vi "Update_WebsocketConnection.vi"(7 "simple_html_chat_ui in":refnum<class "simple_html_chat_ui.lvclass">, 8 "error in (no error)":errorcluster, 11 "WebSocket Connection in":refnum<class "WebSocket Server.lvclass">) -> (0 "error out":errorcluster, 3 "WebSocket Connection out":refnum<class "WebSocket Server.lvclass">, 5 "simple_html_chat_ui out":refnum<class "simple_html_chat_ui.lvclass">)   [LabVIEW 2020, in "simple_html_chat_ui.lvclass"]
uses:
  simple_html_chat_ui.lvclass
  WebSockets-API/Source/WebSockets/WebSocket Server/WebSocket Server.lvclass
  ui/View.vi
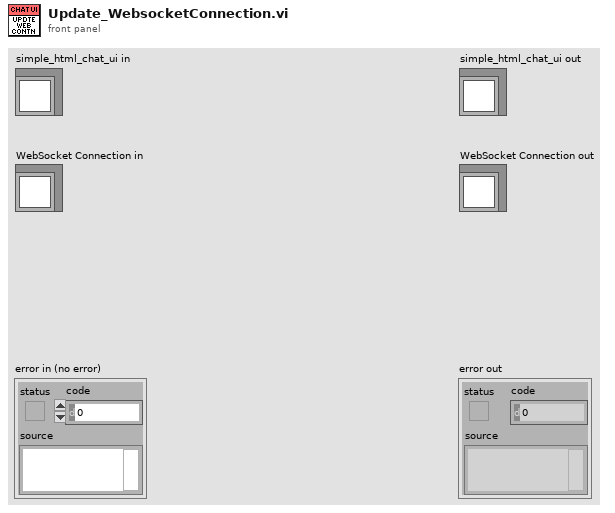
[diagram p1: front panel]
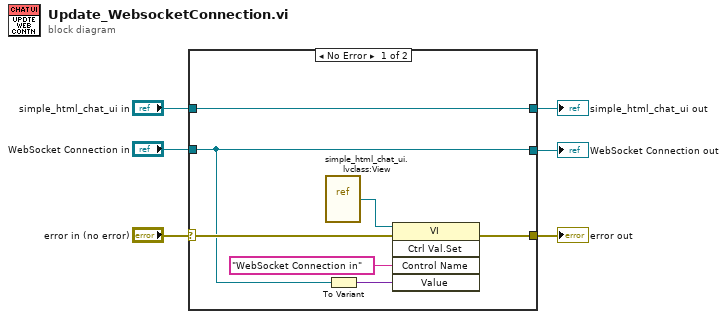
[diagram p0: block diagram]
diagram:
  n1 = case shown="No Error" "error in (no error)" {
    selector: "error in (no error)" -> [w9 w16]
    tunnel: [w8 w16] -> w5
    tunnel: [w13 w15] -> w3
    tunnel: "simple_html_chat_ui in" -> [w13 w15]
    tunnel: "WebSocket Connection in" -> [w7 w14]
    tunnel: [w7 w14] -> w1
    frame No Error {
      n2 = vi-ref "simple_html_chat_ui.lvclass:View.vi"() -> (w10:refnum<vi>)
      n3 = To Variant(anything=w7) -> (Variant=w11:variant)
      n4 = invoke class="VI" method="Ctrl Val.Set"(reference=w10, error in=w9, "Control Name"="WebSocket Connection in", "Value"=w11) -> (error out=w8:errorcluster)  [unwired: 1 in, 4 out]
    }
    frame Error {
    }
  }
  "error out" <- w5
  "simple_html_chat_ui out" <- w3
  "WebSocket Connection out" <- w1
